vi "Support_CreateResults.vi"(0 "Sub test case":string, 1 "Timer start":u32, 2 "Results":T4[](array[typedef]) {"MeasurementValue" format="%.2f"}, 4 "Log":T1[](array[typedef]) {"timestamp" format="%<%H:%M:%S%2u\n%Y/%m/%d>T"}, 5 "error in (no error)":errorcluster, 6 "Invocation info":T2, 8 "Add log to result?":bool, 10 "Test name":string) -> (16 "Pass/fail flag":bool, 17 "Result":string, 18 "Test Data":T3 {"Numeric Measurement" format="%.2f"}, 19 "error out":errorcluster)   [LabVIEW 2009]
doc: "Creates result string."
uses:
  Support_ResultType.ctl
  Support_TestData.ctl
  Support_InvocationInfo.ctl
  Support_LogType.ctl
  <vilib>/addons/_AddQ/G#Object/G#Object.lvclass
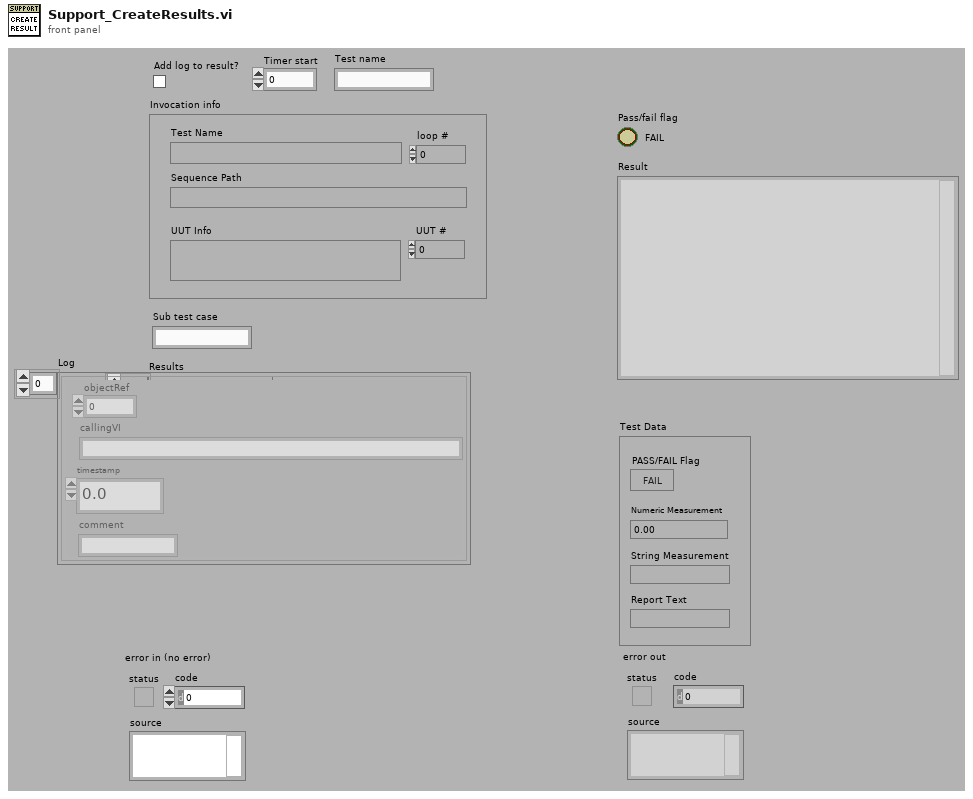
[diagram p1: front panel]
types:
  T1 = typedef "Support_LogType.ctl" = cluster{"objectRef":i32, "callingVI":string, "timestamp":dbl, "comment":string}
  T2 = typedef "Support_InvocationInfo.ctl" = cluster{"UUT #":i32, "loop #":i32, "UUT Info":string, "Test Name":string, "Sequence Path":path}
  T3 = typedef "Support_TestData.ctl" = cluster{"PASS/FAIL Flag":bool, "Numeric Measurement":dbl, "String Measurement":string, "Report Text":string}
  T4 = typedef "Support_ResultType.ctl" = cluster{"Pass":bool, "Comment":string, "MeasurementValue":dbl}
  T5 = enum32{"invalid app kind", "Development System", "Run Time System", "Student Edition", "Embedded LabVIEW", "Evaluation", "Custom"}
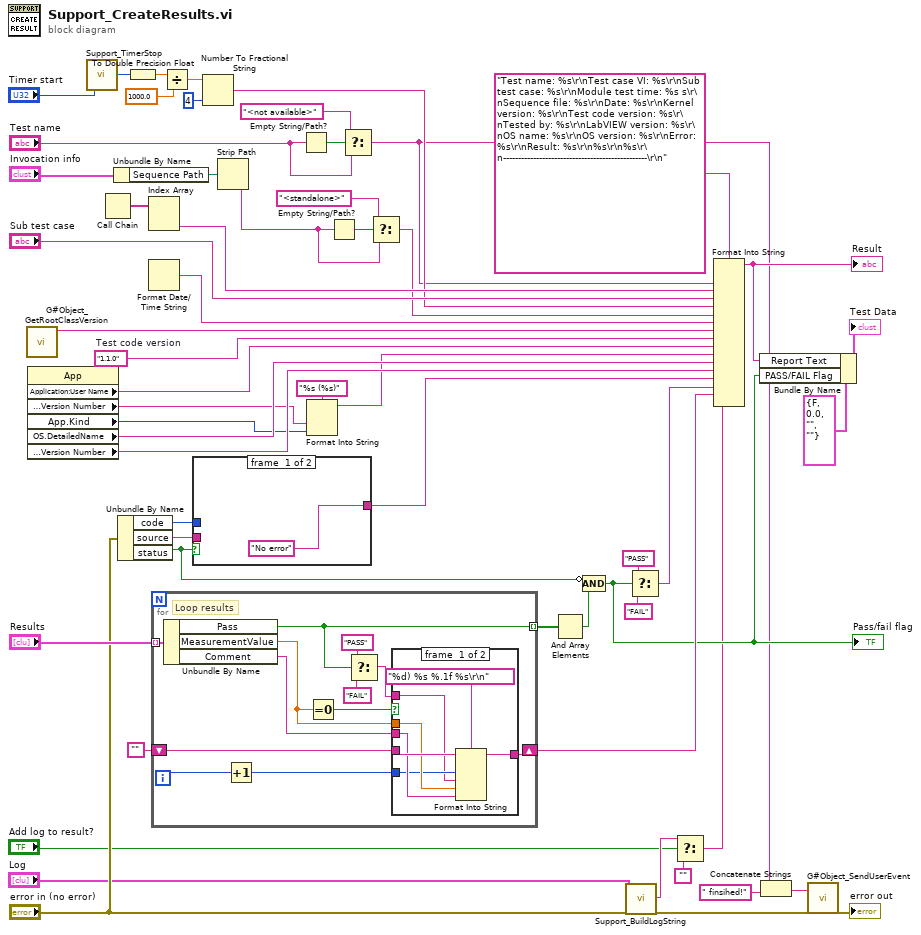
[diagram p0: block diagram]
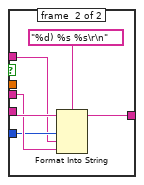
[diagram p2: hidden frame]
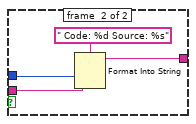
[diagram p3: hidden frame]
diagram:
  w39 = "1.1.0"  # Test code version
  n1 = call <vilib>:"G#Object_GetRootClassVersion.vi"() -> ("version"=w11:string)  [unwired: 18 in, 1 out]
  n2 = property class="App"() -> ("Application:User Name"=w53:string, "Application:Version Number"=w3:string, "App.Kind"=w2:T5, "OS.DetailedName"=w52:string, "Operating System:Version Number"=w51:string)  [unwired: 2 in, 2 out]
  n3 = call "Support_TimerStop.vi"("Start time"="Timer start") -> ("Time (ms)"=w21:u32)  [unwired: 17 in, 1 out]
  n4 = Call Chain() -> (call chain=w57:string[])
  n5 = Unbundle By Name("Invocation info") -> ("Sequence Path"=w37:path)
  n6 = Unbundle By Name("error in (no error)") -> ("code"=w50:i32, "source"=w49:string, "status"=w43:bool)
  n7 = To Double Precision Float(number=w21) -> (double precision float=w19:dbl)
  n8 = Index Array(array=w57) -> (element #2=w36:string)  [unwired: 2 in, 1 out]
  n9 = Format Date/Time String() -> (date/time string=w54:string)  [unwired: 3 in]
  n10 = for {
    tunnel: "Results" -> [w69] mode=indexing
    tunnel: [w59] -> w46 mode=indexing
    shift-right: [w64] -> w44
    shift-left: "" -> [w65]
    i -> [w62]
    # "Loop results"
    n11 = Unbundle By Name(w69) -> ("Pass"=w59:bool, "MeasurementValue"=w67:dbl, "Comment"=w66:string)
    n12 = Increment(x=w62) -> (x+1=w63:i32)
    n13 = Equal To 0?(x=w67) -> (x = 0?=w68:bool)
    n14 = Select(t="PASS", s=w59, f="FAIL") -> (s? t:f=w58:string)
    n15 = case shown="False" w68 {
      tunnel: w67 -> [w72 _]
      tunnel: w66 -> [w73 w79]
      tunnel: w65 -> [w76 w82]
      tunnel: [w75 w81] -> w64
      tunnel: w63 -> [w71 w78]
      tunnel: w58 -> [w70 w77]
      frame #0 {
        n16 = Format Into String(format string="%d) %s %.1f %s\r\n" ("Format String"), initial string=w76, w71, w70, w72, w73) -> (resulting string=w75:string)  [unwired: 1 in, 1 out]
      }
      frame #1 {
        n17 = Format Into String(format string="%d) %s %s\r\n" ("Format String"), initial string=w82, w78, w77, w79) -> (resulting string=w81:string)  [unwired: 1 in, 1 out]
      }
    }
  }
  n18 = Divide(x=w19, y=1000.0) -> (x/y=w18:dbl)
  n19 = case shown="True" w43 {
    tunnel: w50 -> [_ w87]
    tunnel: w49 -> [_ w86]
    tunnel: ["No error" w84] -> w48
    frame #0 {
    }
    frame #1 {
      n20 = Format Into String(format string=" Code: %d Source: %s" ("Format String"), w87, w86) -> (resulting string=w84:string)  [unwired: 2 in, 1 out]
    }
  }
  n21 = Number To Fractional String(number=w18, precision (6)=i16 4) -> (F-format string=w16:string)  [unwired: 2 in]
  n22 = Strip Path(path=w37) -> (name=w13:string)  [unwired: 1 out]
  n23 = Empty String/Path?(string/path="Test name") -> (empty?=w30:bool)
  n24 = Format Into String(format string="%s (%s)", w3, w2) -> (resulting string=w1:string)  [unwired: 2 in, 1 out]
  n25 = Empty String/Path?(string/path=w13) -> (empty?=w14:bool)
  n26 = Select(t="<not available>", s=w30, f="Test name") -> (s? t:f=w6:string)
  n27 = Select(t="<standalone>", s=w14, f=w13) -> (s? t:f=w12:string)
  n28 = And Array Elements(Boolean array=w46) -> (logical AND=w28:bool)
  n29 = Compound Arithmetic op=AND(invert w43, w28) -> (w27:bool)
  "Pass/fail flag" <- w27
  n30 = call "Support_BuildLogString.vi"("log"="Log", "error in (no error)"="error in (no error)") -> ("LogString"=w26:string, "error out"=w10:errorcluster)  [unwired: 16 in]
  n31 = Select(t="PASS", s=w27, f="FAIL") -> (s? t:f=w40:string)
  n32 = Select(t=w26, s="Add log to result?", f="") -> (s? t:f=w24:string)
  n33 = Format Into String(format string="Test name: %s\r\nTest case VI: %s\r\nSub test case: %s\r\nModule test time: %s s\r\nSequence file: %s\r\nDate: %s\r\nKernel version: %s\r\nTest code version: %s\r\nTested by: %s\r\nLabVIEW version: %s\r\nOS name: %s\r\nOS version: %s\r\nError: %s\r\nResult: %s\r\n%s\r\n%s\r\n------------------------------------------------\r\n" ("Format String"), w6, w36, "Sub test case", w16, w12, w54, w11, w39, w53, w1, w52, w51, w48, w40, w44, w24) -> (resulting string=w31:string)  [unwired: 2 in, 1 out]
  "Result" <- w31
  n34 = Bundle By Name(cluster=T3 {"PASS/FAIL Flag"=FALSE, "Numeric Measurement"=0.0, "String Measurement"="", "Report Text"=""} ("Test Data"), "Report Text"=w31, "PASS/FAIL Flag"=w27) -> (→"Test Data":T3)
  n35 = Concatenate Strings(w6, " finsihed!" ("string")) -> (w7:string)
  n36 = call <vilib>:"G#Object_SendUserEvent.vi"("text"=w7, "error in (no error)"=w10) -> ("error out"=→"error out":errorcluster)  [unwired: 16 in, 1 out]
